vi "IO@CheckLogicOn__Parameter.vi"(1 "ParamterIn":string) -> (0 "ParamterOut":string)   [LabVIEW 2020]
panel:
  out "Variable List":string[](array[string])
  in  "Confirm":bool
  in  "Message":string(combo)
  out "IO List":string[](array[string])
  in  "TimeOut":string(combo)
  in  "PortSelect":string(combo)
  # "IO@CheckLogicOn $IOLogic(,$Timeout,[[$label]]$Message)\nIOLogic Express is:\nIO1 & (IO2 | IO3)\nVar==XXX, !=XXX, >=XXX, <=XXX, >XXX, <XXX\nVar <> XXX~YYY, </>XXX~YYY\nVar==NULL, ==EXIST, ==[], ==[;;]\nVar !=NULL, !=EXIST, !=[], !=[;;]\n~IOLogic will inverse Logic\nUse Var@Section to assign which section"
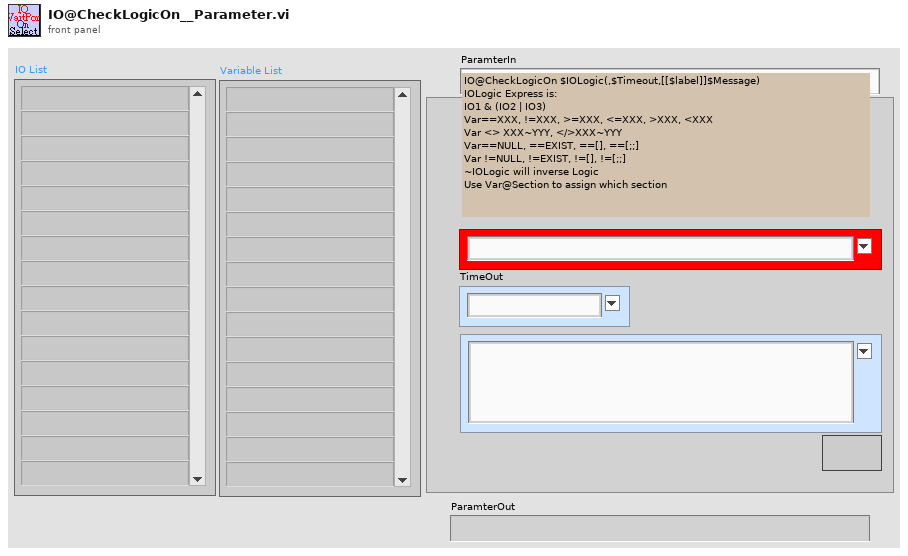
[diagram p1: front panel]
types:
  T1 = enum16{"Get", "Init", "Set", "Delete", "GetElement", "Inc", "Dec", "ReName"}
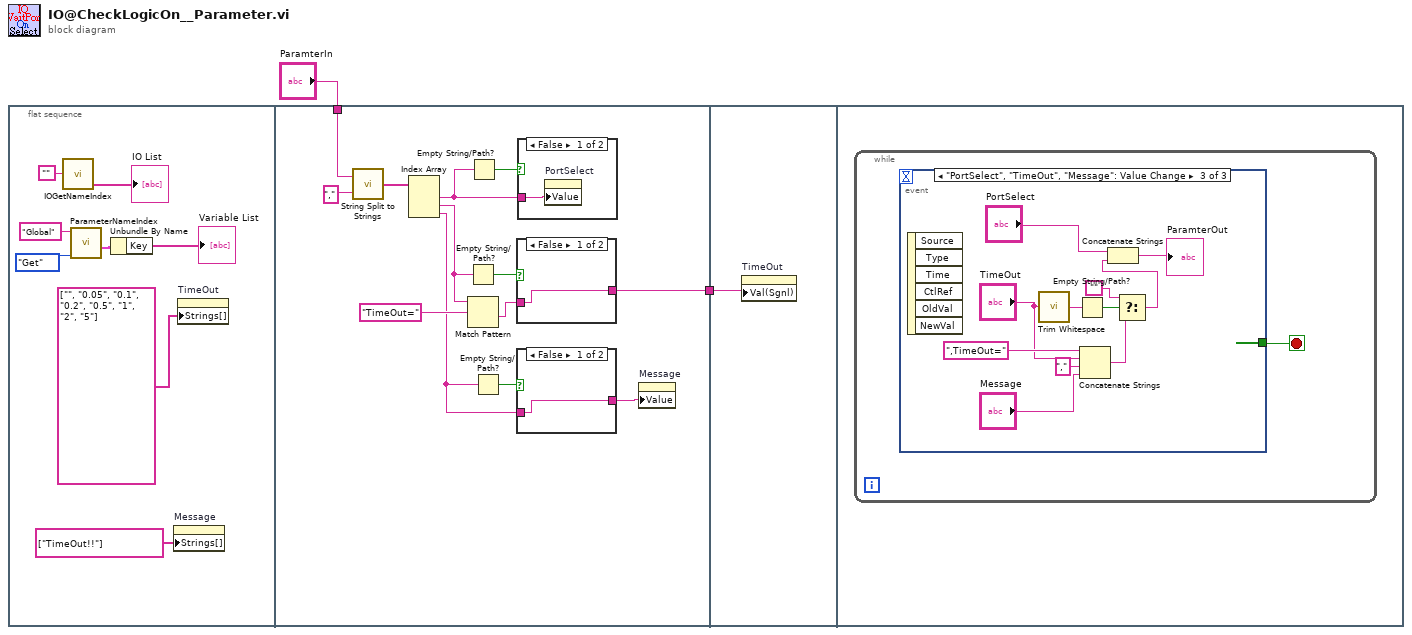
[diagram p0: block diagram]
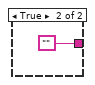
[diagram p2: hidden frame]
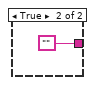
[diagram p3: hidden frame]
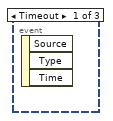
[diagram p5: hidden frame]
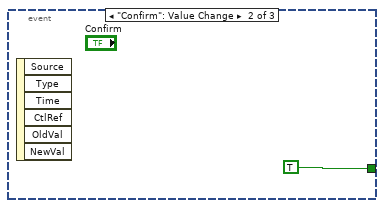
[diagram p6: hidden frame]
diagram:
  n1 = flat-sequence {
    tunnel: "ParamterIn" -> [w22]
    tunnel: [w14] -> w1
    tunnel: w1 -> [w29]
    frame #0 {
      n2 = call "IOGetNameIndex.vi"("PortName"="") -> ("PortNameList Out"=→"IO List":string[])  [unwired: 3 in, 1 out]
      n3 = call "ParameterNameIndex.vi"("OP"=T1."Get", "VariableSection"="Global") -> ("GlobalKeyValue"=w5:cluster{"Key":string[], "Value":string[]})  [unwired: 3 in, 6 out]
      n4 = Unbundle By Name(w5) -> ("Key"=→"Variable List":string[])
      n5 = property on="Message" class="CmbBox"("Strings[]"=string[] ["TimeOut!!"] ("Strings []")) -> ()  [unwired: 2 in, 2 out]
      n6 = property on="TimeOut" class="CmbBox"("Strings[]"=string[] ["", "0.05", "0.1", "0.2", "0.5", "1", "2", "5"] ("Strings []")) -> ()  [unwired: 2 in, 2 out]
    }
    frame #1 {
      n7 = call "String Split to Strings.vi"("search string/char (-)"=",", "String"=w22) -> ("Array"=w21:string[])
      n8 = Index Array(array=w21) -> (element #1=w19:string, element #2=w16:string, element #3=w12:string)  [unwired: 3 in]
      n9 = Empty String/Path?(string/path=w16) -> (empty?=w18:bool)
      n10 = Match Pattern(string=w16, regular expression="TimeOut=") -> (after substring=w17:string)  [unwired: 1 in, 3 out]
      n11 = Empty String/Path?(string/path=w19) -> (empty?=w20:bool)
      n12 = Empty String/Path?(string/path=w12) -> (empty?=w13:bool)
      n13 = case shown="False" w18 {
        tunnel: w17 -> [w26 _]
        tunnel: [w26 ""] -> w14
        frame False {
        }
        frame True {
        }
      }
      n14 = case shown="False" w13 {
        tunnel: w12 -> [w24 _]
        tunnel: [w24 ""] -> w11
        frame False {
        }
        frame True {
        }
      }
      n15 = case shown="False" w20 {
        tunnel: w19 -> [w28 _]
        frame False {
          n16 = property on="PortSelect" class="CmbBox"("Value"=w28) -> ()  [unwired: 2 in, 2 out]
        }
        frame True {
        }
      }
      n17 = property on="Message" class="CmbBox"("Value"=w11) -> ()  [unwired: 2 in, 2 out]
    }
    frame #2 {
      n18 = property on="TimeOut" class="CmbBox"("Val(Sgnl)"=w29) -> ()  [unwired: 2 in, 2 out]
    }
    frame #3 {
      n19 = while {
        stop <- w30 stop-if-true
        n20 = event shown="[2] \"PortSelect\", \"TimeOut\", \"Message\": Value Change" {
          selector: _ -> [_ _ _]
          dyn-events: _ -> [_ _ _]
          timeout: _ -> [_ _ _]
          tunnel: [_ TRUE _] -> w30
          event Timeout {
            n21 = event-data() -> ()  [unwired: 1 in, 3 out]
          }
          event "Confirm": Value Change {
            n22 = event-data() -> ()  [unwired: 1 in, 6 out]
          }
          event "PortSelect", "TimeOut", "Message": Value Change {
            n23 = event-data() -> ()  [unwired: 1 in, 6 out]
            n24 = call <vilib>:"Trim Whitespace.vi"("string"="TimeOut") -> ("trimmed string"=w36:string)  [unwired: 1 in]
            n25 = Empty String/Path?(string/path=w36) -> (empty?=w37:bool)
            n26 = Concatenate Strings(",TimeOut=" ("string"), "TimeOut", "," ("string"), "Message") -> (w39:string)
            n27 = Select(t="", s=w37, f=w39) -> (s? t:f=w34:string)
            n28 = Concatenate Strings("PortSelect", w34) -> (→"ParamterOut":string)
          }
        }
      }
    }
  }
